vi "DrawTextOnImageGreyscale.vi"(4 "Thickness (Default: 1)":i32=1, 5 "Text Drawing Settings (Default: Simplex)":T1={"OpenCV Font Face"=enum."FONT_HERSHEY_SIMPLEX", "Font Scale"=1.0}, 6 "Colour":u8=255, 7 "OpenCV Line Type (Default LINE_8)":T4=enum."LINE_8", 8 "error in (no error)":errorcluster, 9 "Text":string, 10 "Origin":T3, 11 "Greyscale Image":refnum<data-value>) -> (0 "error out":errorcluster, 3 "Greyscale Image (Duplicate)":refnum<data-value>)   [LabVIEW 2020, in "g_ar_toolkit.image.lvlib"]
uses:
  g_ar_toolkit.image.lvlib
  0015c4fc-6a12-4f82-815b-6c2f827f408b.vi
  Line Type.ctl
  Image Point (Fixed).ctl
  Font Face.ctl
  Text Drawing Settings.ctl
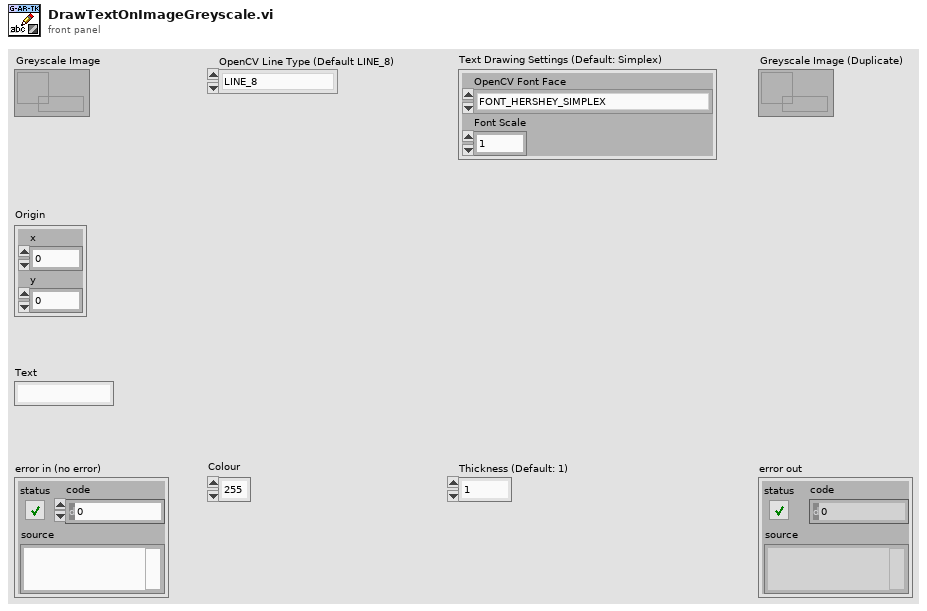
[diagram p1: front panel]
types:
  T1 = typedef "g_ar_toolkit.image.lvlib/Text Drawing Settings.ctl" = cluster{"OpenCV Font Face":T2, "Font Scale":dbl}
  T2 = typedef "g_ar_toolkit.image.lvlib/Font Face.ctl" = enum16{"FONT_HERSHEY_SIMPLEX", "FONT_HERSHEY_PLAIN", "FONT_HERSHEY_DUPLEX", "FONT_HERSHEY_COMPLEX", "FONT_HERSHEY_TRIPLEX", "FONT_HERSHEY_COMPLEX_SMALL", "FONT_HERSHEY_SCRIPT_SIMPLEX", "FONT_HERSHEY_SCRIPT_COMPLEX", "FONT_ITALIC"}
  T3 = typedef "g_ar_toolkit.image.lvlib/Image Point (Fixed).ctl" = cluster{"x":i32, "y":i32}
  T4 = typedef "g_ar_toolkit.image.lvlib/Line Type.ctl" = enum8{"FILLED", "LINE_4", "LINE_8", "LINE_AA"}
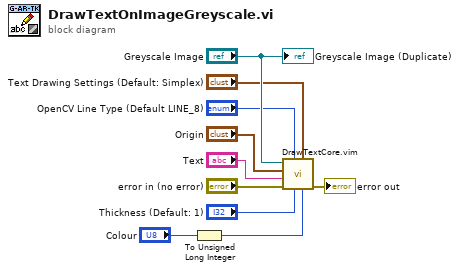
[diagram p0: block diagram]
diagram:
  n1 = To Unsigned Long Integer(number="Colour") -> (unsigned 32bit integer=w1:u32)
  n2 = call "DrawTextCore.vim"("Colour"=w1, "Text Drawing Settings"="Text Drawing Settings (Default: Simplex)", "Thickness"="Thickness (Default: 1)", "OpenCV Line Type"="OpenCV Line Type (Default LINE_8)", "error in (no error)"="error in (no error)", "Text"="Text", "Origin"="Origin", "Src"="Greyscale Image") -> ("error out"=→"error out":errorcluster)  [unwired: 3 in]
  "Greyscale Image (Duplicate)" <- "Greyscale Image"
